vi "CALIBRATE 2016.vi"(0 "flow_slope_IN":dbl=51.35 format="%.2f", 1 "Array in":refnum<k24>[](array[refnum]), 5 "pressure_slope_IN":dbl=23.33 format="%.2f", 7 "Descriptions":string[](array[string]), 9 "string_pot_slope_IN":dbl=1.5 format="%.2f", 11 "error in (no error)":errorcluster, 12 "Sensor Cluster":T1, 14 "Path":path=path "C:/KPRO_2010/Output_files/slopes-cal-record.txt") -> (2 "Array out":refnum<k24>[](array[refnum]), 4 "flow_slope_OUT":dbl=51.35 format="%.2f", 6 "pressure_slope_OUT":dbl=23.33 format="%.2f", 10 "string_pot_slope_OUT":dbl=1.5 format="%.2f", 13 "Sensor Cluster 2":T1, 15 "error out":errorcluster)   [LabVIEW 2016]
uses:
  controls/MCC DAQ Readings.ctl
  C:/Program Files (x86)/National Instruments/LabVIEW 2016/vi.lib/ULx/ULx_LV.dll
  Program Files (x86)/National Instruments/LabVIEW 2016/vi.lib/ULx/ULx_LV.dll
panel:
  out "Loop Counter":i32
  in  "exit":bool
  in  "string_pot":bool
  in  "pressure":bool
  in  "flow":bool
  in  "start path":path=path "C:/"
  in  "all":bool
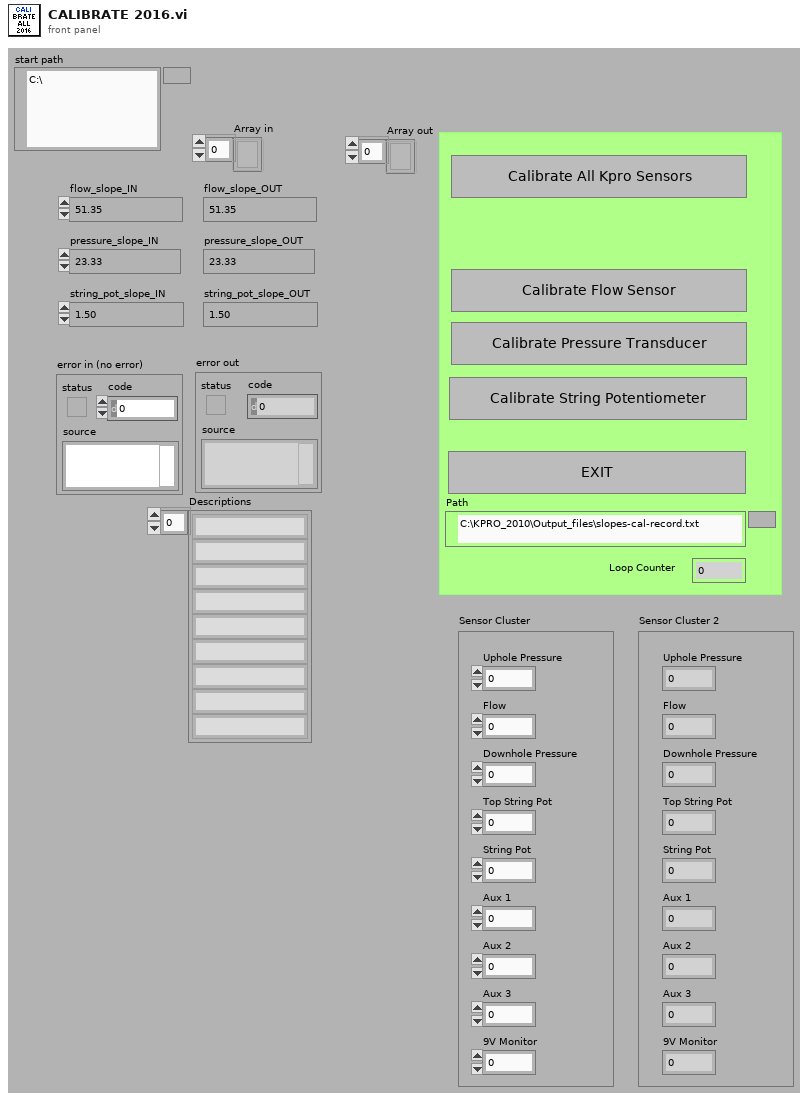
[diagram p1: front panel]
types:
  T1 = typedef "MCC DAQ Readings.ctl" = cluster{"Uphole Pressure":dbl, "Flow":dbl, "Downhole Pressure":dbl, "Top String Pot":dbl, "String Pot":dbl, "Aux 1":dbl, "Aux 2":dbl, "Aux 3":dbl, "9V Monitor":dbl}
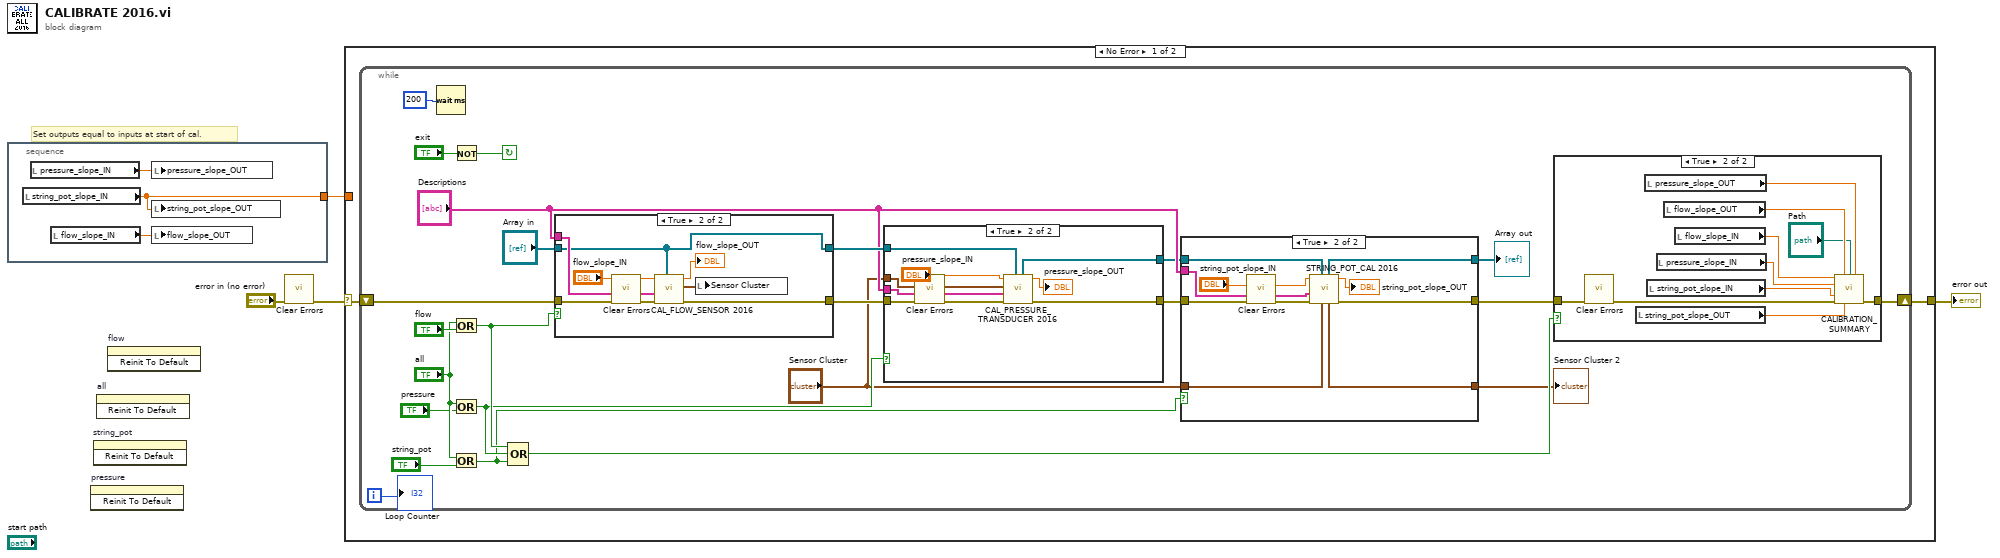
[diagram p0: block diagram]
diagram:
  # "Set outputs equal to inputs at start of cal."
  n1 = stacked-sequence {
    tunnel: [w5] -> w2
    frame #0 {
      n2 = local read "string_pot_slope_IN"() -> (w5:dbl)
      n3 = local read "pressure_slope_IN"() -> (w6:dbl)
      n4 = local read "flow_slope_IN"() -> (w7:dbl)
      n5 = local write "pressure_slope_OUT"(w6) -> ()
      n6 = local write "string_pot_slope_OUT"(w5) -> ()
      n7 = local write "flow_slope_OUT"(w7) -> ()
    }
  }
  n8 = invoke on="pressure" class="Bool" method="Reinit To Default"() -> ()  [unwired: 3 in, 3 out]
  n9 = invoke on="string_pot" class="Bool" method="Reinit To Default"() -> ()  [unwired: 3 in, 3 out]
  n10 = invoke on="all" class="Bool" method="Reinit To Default"() -> ()  [unwired: 3 in, 3 out]
  n11 = invoke on="flow" class="Bool" method="Reinit To Default"() -> ()  [unwired: 3 in, 3 out]
  n12 = call <vilib>:"Clear Errors.vi"("error in (no error)"="error in (no error)") -> ("error out"=w1:errorcluster)  [unwired: 5 in, 1 out]
  n13 = case shown="No Error" w1 {
    selector: w1 -> [w9 w79]
    tunnel: [w8 w79] -> w3
    tunnel: w2 -> [_ _]
    frame No Error {
      n14 = while {
        shift-left: w9 -> [w30]
        shift-right: [w22] -> w8
        i -> [w10]
        stop <- w33 continue-if-true
        n15 = Wait (ms)(milliseconds to wait=u32 200) -> ()  [unwired: 1 out]
        n16 = Not(x="exit") -> (.not. x?=w33:bool)
        n17 = Or(x="all", y="flow") -> (x .or. y?=w21:bool)
        n18 = Or(x="all", y="pressure") -> (x .or. y?=w20:bool)
        n19 = Or(x="all", y="string_pot") -> (x .or. y?=w19:bool)
        n20 = Compound Arithmetic op=OR(w21, w20, w19) -> (w18:bool)
        n21 = case shown="True" w21 {
          tunnel: w30 -> [w70 w78]
          tunnel: [w70 w77] -> w27
          tunnel: "Descriptions" -> [_ w74]
          tunnel: "Array in" -> [w69 w73]
          tunnel: [w69 w73] -> w16
          frame False {
          }
          frame True {
            n22 = call <vilib>:"Clear Errors.vi"("error in (no error)"=w78) -> ("error out"=w71:errorcluster)  [unwired: 5 in, 1 out]
            n23 = call "CAL_FLOW_SENSOR 2016.vi"("Array in"=w73, "error in (no error)"=w71, "Descriptions"=w74, "flow_slope_IN"="flow_slope_IN") -> ("error out"=w77:errorcluster, "Sensor Cluster"=w72:T1, "flow_slope\nmL/min"=→"flow_slope_OUT":dbl)  [unwired: 4 in, 1 out]
            n24 = local write "Sensor Cluster"(w72) -> ()
          }
        }
        n25 = case shown="True" w20 {
          tunnel: [w59 w67] -> w28
          tunnel: w27 -> [w59 w68]
          tunnel: "Sensor Cluster" -> [_ w64]
          tunnel: "Descriptions" -> [_ w63]
          tunnel: w16 -> [w58 w62]
          tunnel: [w58 w61] -> w13
          frame False {
          }
          frame True {
            n26 = call <vilib>:"Clear Errors.vi"("error in (no error)"=w68) -> ("error out"=w60:errorcluster)  [unwired: 5 in, 1 out]
            n27 = call "CAL_PRESSURE_TRANSDUCER 2016.vi"("Array in"=w62, "error in (no error)"=w60, "Descriptions"=w63, "Sensor Cluster"=w64, "pressure_slope_IN"="pressure_slope_IN") -> ("error out"=w67:errorcluster, "pressure_slope_OUT"=→"pressure_slope_OUT":dbl, "Array out"=w61:refnum<k24>[])  [unwired: 3 in, 1 out]
          }
        }
        n28 = case shown="True" w19 {
          tunnel: w28 -> [w47 w51]
          tunnel: [w47 w50] -> w23
          tunnel: "Descriptions" -> [_ w57]
          tunnel: "Sensor Cluster" -> [w46 w56]
          tunnel: w13 -> [w45 w55]
          tunnel: [w45 w54] -> w12
          tunnel: [w46 w49] -> w11
          frame False {
          }
          frame True {
            n29 = call <vilib>:"Clear Errors.vi"("error in (no error)"=w51) -> ("error out"=w48:errorcluster)  [unwired: 5 in, 1 out]
            n30 = call "STRING_POT_CAL 2016.vi"("Sensor Cluster"=w56, "Array in"=w55, "error in (no error)"=w48, "Descriptions"=w57, "string_pot_slope_IN"="string_pot_slope_IN") -> ("error out"=w50:errorcluster, "string_pot_slope_OUT"=→"string_pot_slope_OUT":dbl, "Sensor Cluster 2"=w49:T1, "Array out"=w54:refnum<k24>[])  [unwired: 3 in]
          }
        }
        "Array out" <- w12
        "Sensor Cluster 2" <- w11
        n31 = case shown="True" w18 {
          tunnel: w23 -> [w34 w44]
          tunnel: [w34 w43] -> w22
          frame False {
          }
          frame True {
            n32 = call <vilib>:"Clear Errors.vi"("error in (no error)"=w44) -> ("error out"=w35:errorcluster)  [unwired: 5 in, 1 out]
            n33 = local read "string_pot_slope_OUT"() -> (w37:dbl)
            n34 = local read "pressure_slope_OUT"() -> (w42:dbl)
            n35 = local read "string_pot_slope_IN"() -> (w38:dbl)
            n36 = local read "pressure_slope_IN"() -> (w39:dbl)
            n37 = local read "flow_slope_OUT"() -> (w41:dbl)
            n38 = local read "flow_slope_IN"() -> (w40:dbl)
            n39 = call "CALIBRATION_SUMMARY.vi"("flow_slope_IN"=w40, "flow_slope_OUT"=w41, "Path"="Path", "pressure_slope_OUT"=w42, "pressure_slope_IN"=w39, "string_pot_slope_IN"=w38, "error in (no error)"=w35, "string_pot_slope_OUT"=w37) -> ("error out"=w43:errorcluster)  [unwired: 7 in]
          }
        }
        "Loop Counter" <- w10
      }
    }
    frame Error {
    }
  }
  "error out" <- w3
